vi "dotNET timestamp to LV timestamp.vi"(10 "seconds since epoch":i64, 11 "positive fractions of a second":u64) -> (3 "t0":timestamp)   [LabVIEW 2020, in "NI_VS Waveform Streaming Interface.lvlib"]
uses:
  NI_VS Waveform Streaming Interface.lvlib
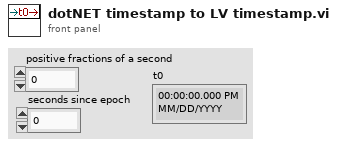
[diagram p1: front panel]
types:
  T1 = cluster{"seconds since epoch":i64, "positive fractions of a second":u64}
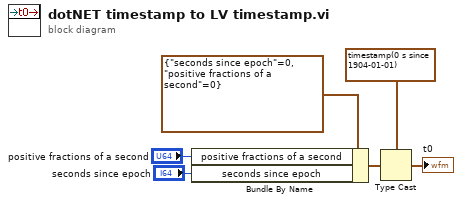
[diagram p0: block diagram]
diagram:
  n1 = Bundle By Name(cluster=T1 {"seconds since epoch"=0, "positive fractions of a second"=0}, "positive fractions of a second"="positive fractions of a second", "seconds since epoch"="seconds since epoch") -> (w5:T1)
  n2 = Type Cast(type=timestamp(0 s since 1904-01-01) ("t0"), x=w5) -> (*(type *) &x=→"t0":timestamp)
